vi "PH_gentec_M-Link.Action Measure.vi"(0 "VI in":refnum<vi>, 5 "error in (no error)":errorcluster) -> (14 "VI out":refnum<vi>, 19 "error out":errorcluster)   [LabVIEW 2014, in "PH_gentec_M-Link.lvlib"]
uses:
  PH_gentec_M-Link.lvlib
  PH_Powermeter_BaseClass/PH_Powermeter_BaseClass.State.ctl
  non_GPL/instr.lib/gentec-M-LINK/gentec-M-Link - Driver.lvlib
  PH_Powermeter_BaseClass/PH_Powermeter_BaseClass.lvlib
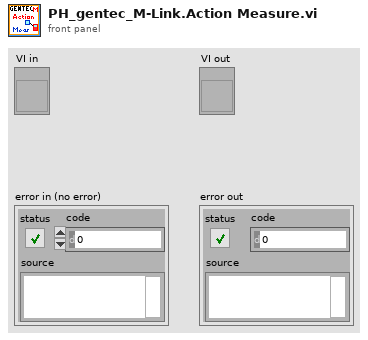
[diagram p1: front panel]
types:
  T1 = typedef "PH_Powermeter_BaseClass.lvlib/PH_Powermeter_BaseClass.State.ctl" = enum32{"off", "operating", "opened", "checked", "connected", "Sets to change", "running"}
  T2 = typedef "PH_Powermeter_BaseClass.lvlib/PH_Powermeter_BaseClass.i attribute.ctl" = cluster{"GUI References":T3, "Connection":T4, "Head Attributes":T5, "VISA resource":refnum<visa-resource-name>, "Energy":T6, "Service ID Energy":i32, "Wanted Settings":T7, "Current Settings":T7}
  T3 = typedef "PH_Powermeter_BaseClass.lvlib/PH_Powermeter_BaseClass.GUI Refs.ctl" = cluster{"Head Attributes":refnum<vi>, "Energy":refnum<vi>, "Connection":refnum<vi>, "VISA Resource":refnum<vi>, "Energy evolution":refnum<vi>, "Scaling Factor":refnum<vi>, "Range":refnum<vi>, "Wavelength":refnum<vi>, "Trigger Level":refnum<vi>, "Wanted Settings":refnum<vi>, "Current Settings":refnum<vi>}
  T4 = typedef "PH_Powermeter_BaseClass.lvlib/PH_Powermeter_BaseClass.Connection.ctl" = cluster{"failed checks":i8, "Timeout":bool, "Data read":string, "Failure":bool, "Error":bool, "State":T1}
  T5 = typedef "PH_Powermeter_BaseClass.lvlib/PH_Powermeter_BaseClass.Head Attributes.ctl" = cluster{"Instrument Type":string, "Head Version":string, "Head Name":string, "Serial Number":string, "Firmware":string, "Sensor Type":string, "MinimumRange":u32, "Maximum Range":u32, "Min Wavelength":i32, "Max Wavelength":i32}
  T6 = typedef "PH_Powermeter_BaseClass.lvlib/PH_Powermeter_BaseClass.Energy.ctl" = cluster{"current Value":dbl, "unscaled":dbl, "Scaling Factor":dbl}
  T7 = typedef "PH_Powermeter_BaseClass.lvlib/PH_gentec_BaseClass.Head Settings.ctl" = cluster{"Trigger Level":dbl, "Wavelength":u32, "Range":u32}
  T8 = typedef "PH_gentec_M-Link.lvlib/PH_gentec_M-Link.i attribute.ctl" = cluster{"GUI References":cluster{"Wanted Head Settings":refnum<vi>, "Current Head Settings":refnum<vi>, "Set Auto Range":refnum<vi>, "Trigger Polarity":refnum<vi>, "Trigger Source":refnum<vi>, "Waveform Averages":refnum<vi>, "Continuous":refnum<vi>, "get one Value":refnum<vi>}, "Wanted Head Settings":T9, "Current Head Settings":T9}
  T9 = typedef "PH_gentec_M-Link.lvlib/PH_gentec_M-Link.Head Settings.ctl" = cluster{"Measurement Mode":T10, "Enable Anticipation":bool, "Set Auto Range":bool, "Block Signal":bool, "Set Head Attenuator":bool, "Enable SSE":bool, "Trigger Polarity":T11, "Trigger Source":T12, "Waveform Averages":T13, "Set Zero":i32, "Current Measurement":i32, "Start Data Flow":bool}
  T10 = typedef "gentec-M-Link - Driver.lvlib/gentec-M-Link.Measurement Mode.ctl" = u16
  T11 = typedef "gentec-M-Link - Driver.lvlib/gentec-M-Link.Trigger Polarity.ctl" = u16
  T12 = typedef "gentec-M-Link - Driver.lvlib/gentec-M-Link.Trigger Source.ctl" = u16
  T13 = typedef "gentec-M-Link - Driver.lvlib/gentec-M-Link.Waveform Averages.ctl" = u16
  T14 = typedef "gentec-M-Link - Driver.lvlib/gentec-M-Link.Range.ctl" = u16
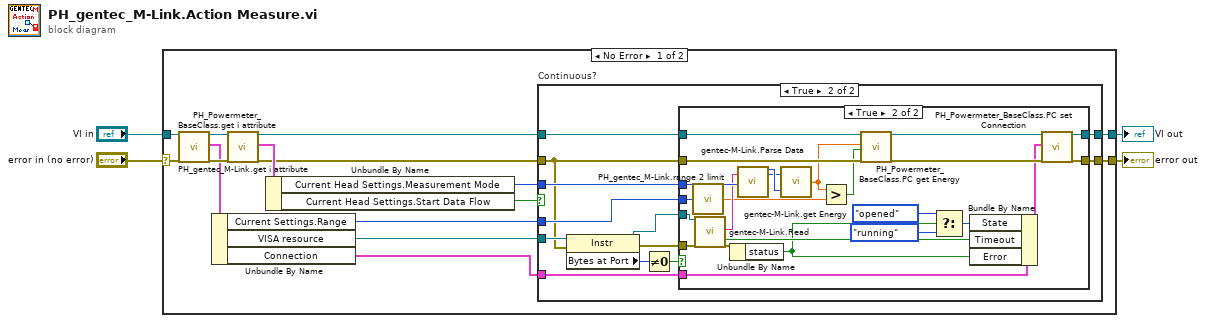
[diagram p0: block diagram]
diagram:
  n1 = case shown="No Error" "error in (no error)" {
    selector: "error in (no error)" -> [w6 w60]
    tunnel: [w14 w61] -> w4
    tunnel: [w13 w60] -> w3
    tunnel: "VI in" -> [w11 w61]
    frame No Error {
      n2 = call "PH_Powermeter_BaseClass.get i attribute.vi"("i ref in"=w11, "error in (no error)"=w6) -> ("i ref out"=w10:refnum<vi>, "i attribute"=w9:T2, "error out"=w12:errorcluster)  [unwired: 15 in]
      n3 = Unbundle By Name(w9) -> ("Current Settings.Range"=w5:u32, "VISA resource"=w8:refnum<visa-resource-name>, "Connection"=w7:T4)
      n4 = call "PH_gentec_M-Link.get i attribute.vi"("i ref in"=w10, "error in (no error)"=w12) -> ("i ref out"=w17:refnum<vi>, "i attribute"=w18:T8, "error out"=w16:errorcluster)  [unwired: 15 in]
      n5 = Unbundle By Name(w18) -> ("Current Head Settings.Measurement Mode"=w19:T10, "Current Head Settings.Start Data Flow"=w15:bool)
      n6 = case "Continuous?" shown="True" w15 {
        tunnel: w17 -> [w21 w26]
        tunnel: [w21 w24] -> w14
        tunnel: w16 -> [w20 w25]
        tunnel: [w20 w23] -> w13
        tunnel: w8 -> [_ w29]
        tunnel: w19 -> [_ w28]
        tunnel: w5 -> [_ w27]
        tunnel: w7 -> [_ w22]
        frame False {
        }
        frame True {
          n7 = property class="Instr"(reference=w29, error in=w25) -> (reference out=w31:refnum<visa-resource-name>, error out=w30:errorcluster, "Bytes at Port"=w33:u32)
          n8 = Not Equal To 0?(x=w33) -> (x != 0?=w32:bool)
          n9 = case shown="True" w32 {
            tunnel: w31 -> [_ w59]
            tunnel: w30 -> [_ w58]
            tunnel: w28 -> [_ w57]
            tunnel: w25 -> [w35 w53]
            tunnel: [w35 w44] -> w23
            tunnel: w26 -> [w34 w52]
            tunnel: [w34 w46] -> w24
            tunnel: w27 -> [_ w48]
            tunnel: w22 -> [_ w43]
            frame False {
            }
            frame True {
              n10 = call "PH_gentec_M-Link.range 2 limit.vi"("Range"=w48) -> ("limit"=w50:dbl)
              n11 = call "gentec-M-Link.Read.vi"("VISA resource (In)"=w59, "error in (no error)"=w58) -> ("Data Read"=w56:string, "Read Timeout"=w41:bool, "error out"=w40:errorcluster)  [unwired: 13 in, 2 out]
              n12 = Unbundle By Name(w40) -> ("status"=w39:bool)
              n13 = call "gentec-M-Link.Parse Data.vi"("Data Bytes"=w56, "Measurement"=w57) -> ("ADC Counts"=w55:u16, "Range"=w54:T14)  [unwired: 13 in, 3 out]
              n14 = call "gentec-M-Link.get Energy.vi"("ADC Counts"=w55, "Range"=w54) -> ("Energy [J]"=w51:dbl)
              n15 = Greater?(x=w51, y=w50) -> (0:w49:bool)
              n16 = call "PH_Powermeter_BaseClass.PC get Energy.vi"("i ref in"=w52, "unscaled Energy [J]"=w51, "Out of range?"=w49, "error in"=w53) -> ("i ref out"=w47:refnum<vi>, "error out"=w45:errorcluster)  [unwired: 14 in]
              n17 = Select(t=PH_Powermeter_BaseClass.State."opened", s=w39, f=PH_Powermeter_BaseClass.State."running" ("State")) -> (s? t:f=w37:T1)
              n18 = Bundle By Name(cluster=w43, "State"=w37, "Timeout"=w41, "Error"=w39) -> (w42:T4)
              n19 = call "PH_Powermeter_BaseClass.PC set Connection.vi"("VI in"=w47, "Connection"=w42, "error in (no error)"=w45) -> ("VI out"=w46:refnum<vi>, "error out"=w44:errorcluster)  [unwired: 15 in]
            }
          }
        }
      }
    }
    frame Error {
    }
  }
  "VI out" <- w4
  "error out" <- w3
